vi "xmlEditforHW.vi"(0 "属性新值":string[](array[string]), 3 "属性索引":dbl[](array[numeric]), 4 "tagID":string="Outcome", 5 "xml路径":path) -> (1 "saved?":bool, 2 "loaded":bool)   [LabVIEW 2011]
panel:
  out "错误输出":errorcluster
  in  "错误输入":errorcluster
  in  "MSXML2.IXMLDOMDocument2":refnum<k7>
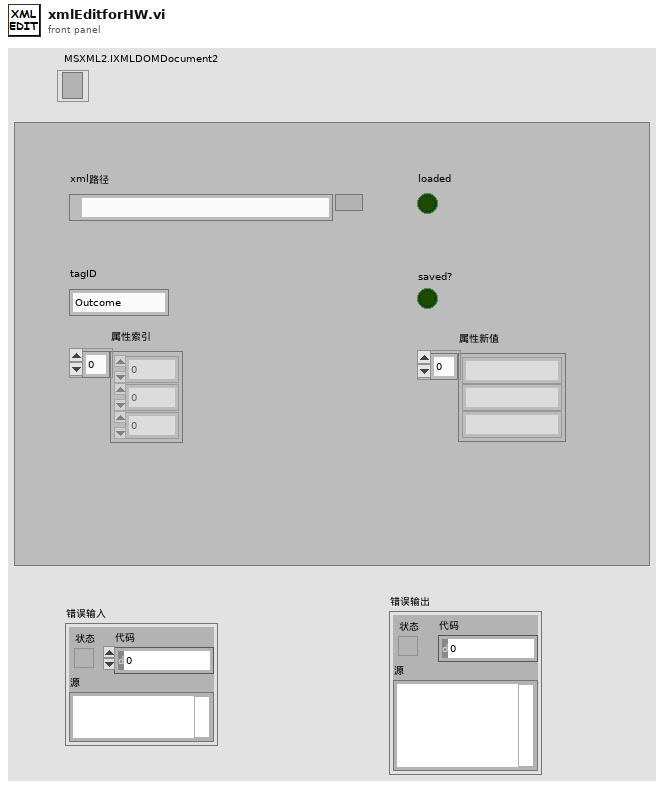
[diagram p1: front panel]
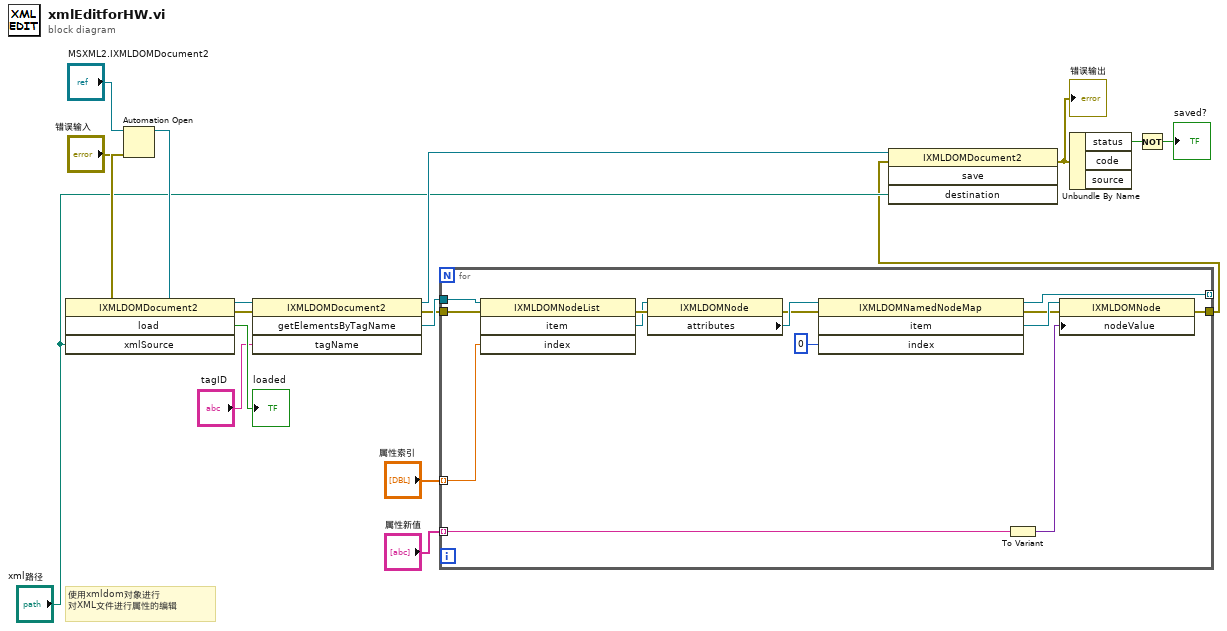
[diagram p0: block diagram]
diagram:
  # "使用xmldom对象进行\n对XML文件进行属性的编辑"
  n1 = Automation Open(error in (no error)="错误输入", Automation Refnum="MSXML2.IXMLDOMDocument2") -> (Automation Refnum=w17:refnum<k7>, error out=w14:errorcluster)  [unwired: 2 in]
  n2 = invoke class="IXMLDOMDocument2" method="load"(reference=w17, error in=w14, "xmlSource"="xml路径") -> (reference out=w15:refnum<k7>, error out=w13:errorcluster, "load"=→"loaded":bool)  [unwired: 1 in, 1 out]
  n3 = invoke class="IXMLDOMDocument2" method="getElementsByTagName"(reference=w15, error in=w13, "tagName"="tagID") -> (reference out=w12:refnum<k7>, error out=w1:errorcluster, "getElementsByTagName"=w2:refnum<k7>)  [unwired: 1 in, 1 out]
  n4 = for {
    tunnel: "属性索引" -> [w21] mode=indexing
    tunnel: "属性新值" -> [w30] mode=indexing
    tunnel: [w28] -> _ mode=indexing
    tunnel: [w27] -> w3
    tunnel: w2 -> [w20]
    tunnel: w1 -> [w19]
    n5 = invoke class="IXMLDOMNodeList" method="item"(reference=w20, error in=w19, "index"=w21) -> (error out=w25:errorcluster, "item"=w24:refnum<k7>)  [unwired: 1 in, 2 out]
    n6 = property class="IXMLDOMNode"(reference=w24, error in=w25) -> (error out=w22:errorcluster, "attributes"=w23:refnum<k7>)  [unwired: 1 out]
    n7 = invoke class="IXMLDOMNamedNodeMap" method="item"(reference=w23, error in=w22, "index"=0) -> (reference out=w28:refnum<k7>, error out=w31:errorcluster, "item"=w32:refnum<k7>)  [unwired: 1 in, 1 out]
    n8 = To Variant(anything=w30) -> (Variant=w29:variant)
    n9 = property class="IXMLDOMNode"(reference=w32, error in=w31, "nodeValue"=w29) -> (error out=w27:errorcluster)  [unwired: 1 out]
  }
  n10 = invoke class="IXMLDOMDocument2" method="save"(reference=w12, error in=w3, "destination"="xml路径") -> (error out=w9:errorcluster)  [unwired: 1 in, 3 out]
  "错误输出" <- w9
  n11 = Unbundle By Name(w9) -> ("status"=w8:bool)  [unwired: 2 out]
  n12 = Not(x=w8) -> (.not. x?=→"saved?":bool)
